vi "PopulateTestTree.vi"(8 "error in (no error)":errorcluster, 10 "Test Configuration":T1, 11 "TreeControl in":refnum<vi>) -> (0 "error out":errorcluster, 1 "All Test Tree Tags":string[](array[string]))   [LabVIEW 2018]
uses:
  TestConfiguration.ctl
  Tree/Controls/Plugins Tree Item Type.ctl
  NistPluggableModules/TestClass/Test.lvclass
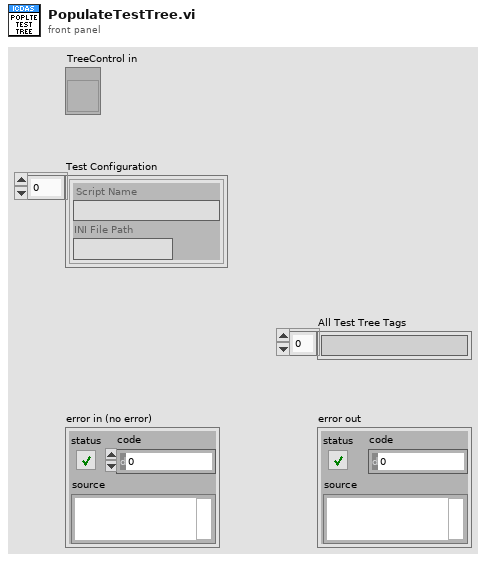
[diagram p1: front panel]
types:
  T1 = typedef "TestConfiguration.ctl" = cluster{"Script Name":string, "INI File Path":string}[]
  T2 = typedef "Plugins Tree Item Type.ctl" = enum16{"Plugin", "Instrument", "INI File", "INI Script"}
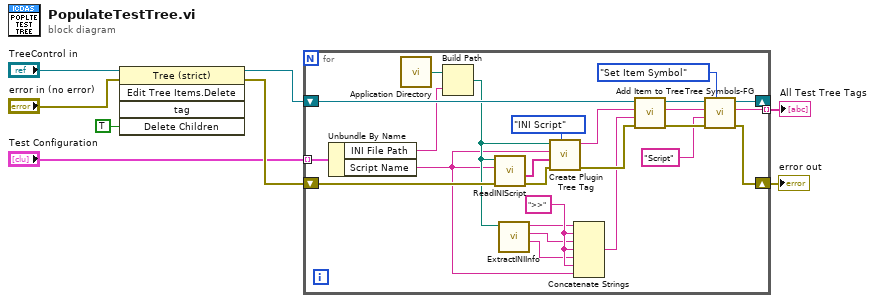
[diagram p0: block diagram]
diagram:
  n1 = invoke class="Tree (strict)" method="Edit Tree Items.Delete"(reference="TreeControl in", error in="error in (no error)", "Delete Children"=TRUE ("Delete Children?")) -> (reference out=w5:refnum<vi>, error out=w7:errorcluster)  [unwired: 2 in, 3 out]
  n2 = for {
    tunnel: "Test Configuration" -> [w33] mode=indexing
    shift-right: [w21] -> w4
    shift-left: w7 -> [w32]
    shift-right: [w20] -> _
    shift-left: w5 -> [w29]
    tunnel: [w10] -> w1 mode=indexing
    w17 = ">>" ("Module Name")
    n3 = Unbundle By Name(w33) -> ("INI File Path"=w18:string, "Script Name"=w11:string)
    n4 = call <vilib>:"Application Directory.vi"() -> ("Application Directory"=w19:path)
    n5 = Build Path(base path=w19, name or relative path=w18) -> (appended path=w13:path)
    n6 = call "ReadINIScript.vi"("error in (no error)"=w32, "Script Name"=w11, "INI File Path"=w13) -> ("error out"=w31:errorcluster, "Script with $"=w9:string[])  [unwired: 5 in, 2 out]
    n7 = call "ExtractINIInfo.vi"("INI File Path"=w13) -> ("INI File Name"=w16:string, "Instrument name"=w15:string, "Module Name"=w14:string)  [unwired: 5 in, 3 out]
    n8 = call "Create Plugin Tree Tag.vi"("ItemType"=Plugins_Tree_Item_Type."INI Script", "error in (no error)"=w31, "Script"=w9, "Name"=w11, "VISA Resource"=w13) -> ("error out"=w28:errorcluster, "Tag"=w27:string)  [unwired: 4 in, 1 out]
    n9 = Concatenate Strings(w14, w17, w15, w17, w16, w17, w11) -> (w12:string)
    n10 = call "Add Item to Tree.vi"("error in (no error)"=w28, "Item Name"=w12, "Item Tag"=w27, "Tree Ref"=w29) -> ("error out"=w26:errorcluster, "Item Tag out"=w25:string, "reference out"=w24:refnum<vi>)  [unwired: 4 in, 1 out]
    n11 = call "Tree Symbols-FG.vi"("Actions"=enum16{"Init Symbols", "Set Item Symbol"}."Set Item Symbol", "error in (no error)"=w26, "Symbol Name"="Script", "Item Tag"=w25, "Tree Ref"=w24) -> ("error out"=w21:errorcluster, "Item Tag out"=w10:string, "Tree Ref out"=w20:refnum<vi>)  [unwired: 4 in]
  }
  "error out" <- w4
  "All Test Tree Tags" <- w1
